vi "Read Analog Input.vi"(0 "Control":T1, 3 "input terminal configuration":i32(ring)=10083 items=["default"=-1, "RSE"=10083, "NRSE"=10078, "Differential"=10106, "Pseudodifferential"=12529], 5 "error in":errorcluster, 6 "Device Name":string="Dev2") -> (14 "data":dbl format="%.4f", 19 "error out":errorcluster={"status"=TRUE, "code"=-200220, "source"="DAQmx Create Channel (DO-Digital Output).vi:2<append>\n<B>Device Specified: </B>Dev1\n\n<B>Task Name: </B>_unnamedTask<0>"})   [LabVIEW 2015]
uses:
  Analog Inputs.ctl
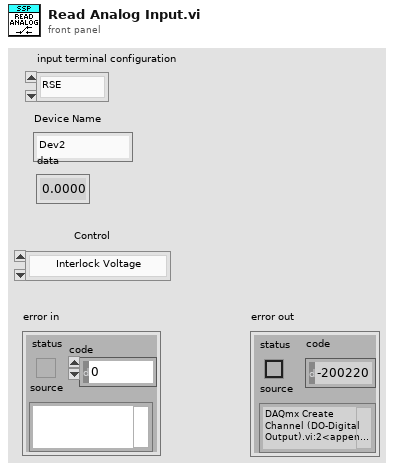
[diagram p1: front panel]
types:
  T1 = typedef "Analog Inputs.ctl" = enum16{"Interlock Voltage"}
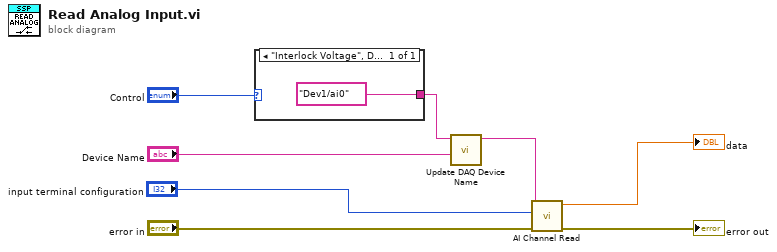
[diagram p0: block diagram]
diagram:
  n1 = case shown="\"Interlock Voltage\", Default" "Control" {
    tunnel: ["Dev1/ai0"] -> w7
    frame "Interlock Voltage", Default {
    }
  }
  n2 = call "Update DAQ Device Name.vi"("Device Name"="Device Name", "Lines in (String)"=w7) -> ("Lines out (DAQmx Physical Channels)"=w3:tag)  [unwired: 9 in]
  n3 = call "AI Channel Read.vi"("error in"="error in", "input terminal configuration"="input terminal configuration", "physical channels"=w3) -> ("error out"=→"error out":errorcluster, "data"=→"data":dbl)  [unwired: 7 in]
